vi "SVN_ls.vi"(6 "password":string, 7 "username":string, 8 "error in (no error)":errorcluster, 11 "URL":string) -> (0 "error out":errorcluster, 2 "lastChangeDate":string, 3 "Items":string[](array[string]))   [LabVIEW 2017]
panel:
  out "Command":string
  out "standard output":string
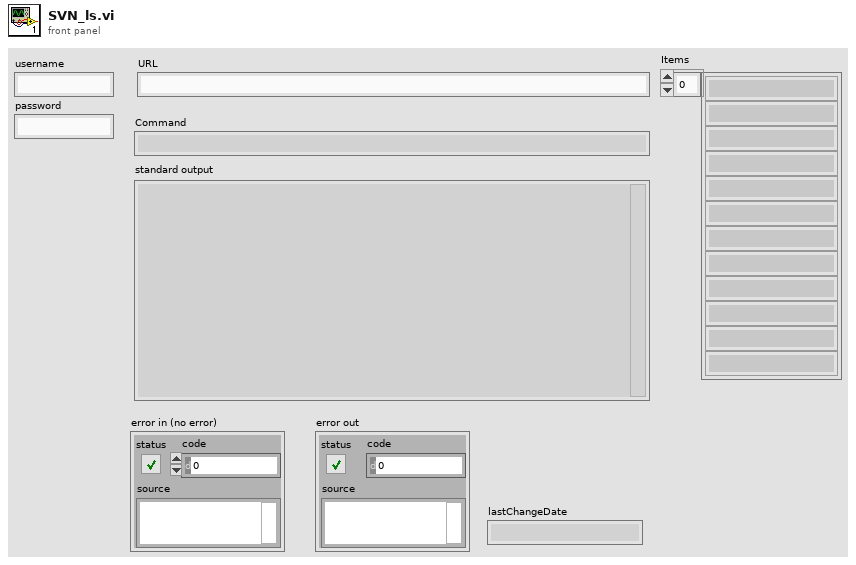
[diagram p1: front panel]
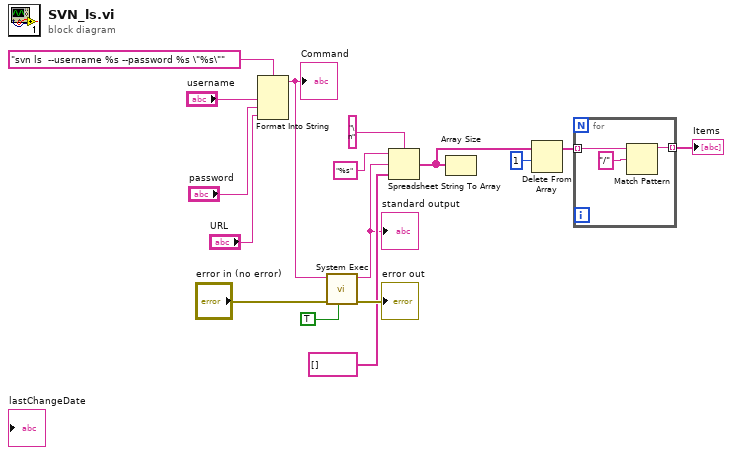
[diagram p0: block diagram]
diagram:
  n1 = Format Into String(format string="svn ls  --username %s --password %s \"%s\"" ("command line"), "username", "password", "URL") -> (resulting string=w12:string)  [unwired: 2 in, 1 out]
  "Command" <- w12
  n2 = call <vilib>:"System Exec.vi"("run minimized? (F)"=TRUE, "error in (no error)"="error in (no error)", "command line"=w12) -> ("error out"=→"error out":errorcluster, "standard output"=w7:string)  [unwired: 5 in, 2 out]
  "standard output" <- w7
  n3 = Spreadsheet String To Array(delimiter (Tab)="\n", format string="%s", spreadsheet string=w7, array type (2D Dbl)=string[] []) -> (array=w3:string[])
  n4 = Array Size(array=w3) -> ()  [unwired: 1 out]
  n5 = Delete From Array(array=w3, length=1) -> (array with subset deleted=w1:string[])  [unwired: 1 in, 1 out]
  n6 = for {
    tunnel: w1 -> [w19] mode=indexing
    tunnel: [w17] -> w4 mode=indexing
    n7 = Match Pattern(string=w19, regular expression="/") -> (before substring=w17:string)  [unwired: 1 in, 3 out]
  }
  "Items" <- w4
